vi "Create Instance.vi"(8 "error in (no error)":errorcluster, 10 "Configuration":T1) -> (0 "error out":errorcluster, 3 "Power Meter out":refnum<class "Power Meter.lvclass">)   [LabVIEW 2023, in "Power Meter.lvlib" / "Power Meter.lvclass"]
uses:
  Power Meter.lvclass
  Power Meter.lvclass/Power Meter.ctl
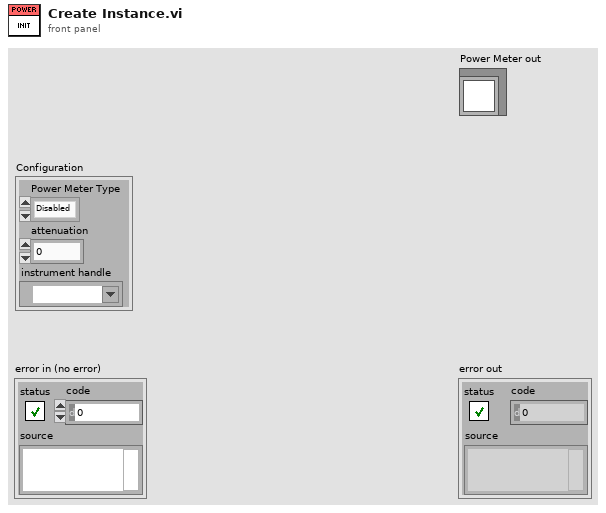
[diagram p1: front panel]
types:
  T1 = cluster{"Power Meter Type":enum16{"Disabled", "Thorlabs", "Newport", "Coherent"}, "attenuation":dbl, "instrument handle":refnum<visa-resource-name>}
  T2 = enum16{"Disabled", "Thorlabs", "Newport", "Coherent"}
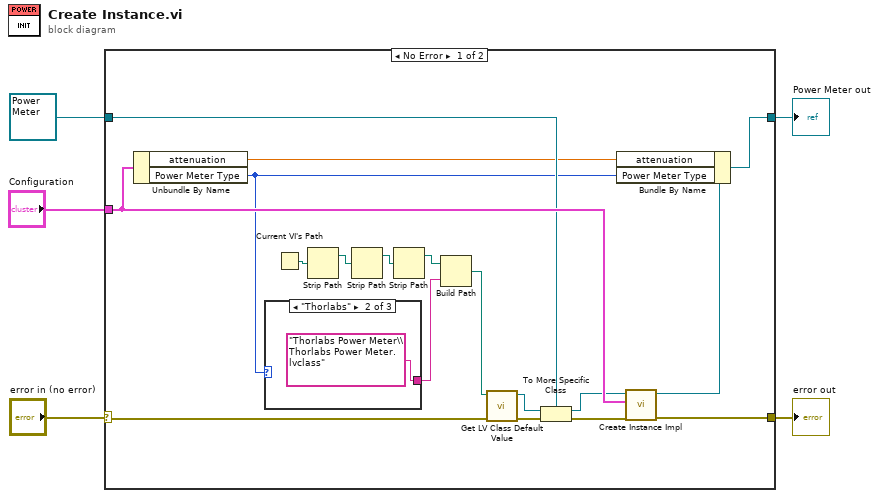
[diagram p0: block diagram]
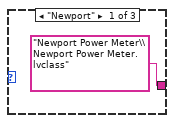
[diagram p2: hidden frame]
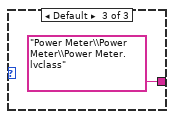
[diagram p3: hidden frame]
diagram:
  n1 = case shown="No Error" "error in (no error)" {
    selector: "error in (no error)" -> [w18 w28]
    tunnel: [w23 w28] -> w4
    tunnel: [w9 w27] -> w2
    tunnel: refnum<class "Power Meter.lvclass"> refnum ("Power Meter in") -> [w10 w27]
    tunnel: "Configuration" -> [w22 _]
    frame No Error {
      n2 = Unbundle By Name(w22) -> ("attenuation"=w7:dbl, "Power Meter Type"=w6:T2)
      n3 = case shown="\"Thorlabs\"" w6 {
        tunnel: ["Newport Power Meter\\Newport Power Meter.lvclass" "Thorlabs Power Meter\\Thorlabs Power Meter.lvclass" "Power Meter\\Power Meter\\Power Meter.lvclass"] -> w21
        frame "Newport" {
        }
        frame "Thorlabs" {
        }
        frame Default {
        }
      }
      n4 = Current VI's Path() -> (path=w20:path)
      n5 = Strip Path(path=w20) -> (stripped path=w19:path)  [unwired: 1 out]
      n6 = Strip Path(path=w19) -> (stripped path=w12:path)  [unwired: 1 out]
      n7 = Strip Path(path=w12) -> (stripped path=w11:path)  [unwired: 1 out]
      n8 = Build Path(base path=w11, name or relative path=w21) -> (appended path=w13:path)
      n9 = call <vilib>:"Get LV Class Default Value.vi"("error in (no error)"=w18, "class path"=w13) -> ("error out"=w17:errorcluster, "object"=w15:refnum<class>)  [unwired: 8 in]
      n10 = To More Specific Class(target class=w10, reference=w15, error in=w17) -> (specific class reference=w14:refnum<class "Power Meter.lvclass">, error out=w16:errorcluster)
      n11 = call-dynamic "Create Instance Impl.vi"("error in (no error)"=w16, "Configuration"=w22, "Power Meter in"=w14) -> ("error out"=w23:errorcluster, "Power Meter out"=w8:refnum<class "Power Meter.lvclass">)  [unwired: 7 in]
      n12 = Bundle By Name(cluster=w8, "attenuation"=w7, "Power Meter Type"=w6) -> (w9:refnum<class "Power Meter.lvclass">)
    }
    frame Error {
    }
  }
  "error out" <- w4
  "Power Meter out" <- w2
